vi "Get Command Bits.vi"(8 "error in (no error)":errorcluster, 11 "RFFE RegWrite Command in":refnum<class "RFFE RegWrite Command.lvclass">) -> (0 "error out":errorcluster, 2 "Command Bits":u8[](array[numeric]) format="%02x", 3 "RFFE RegWrite Command out":refnum<class "RFFE RegWrite Command.lvclass">)   [LabVIEW 2018, in "MIPI RFFE API.lvlib" / "RFFE RegWrite Command.lvclass"]
uses:
  RFFE RegWrite Command.lvclass
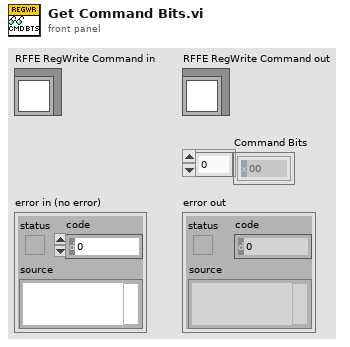
[diagram p1: front panel]
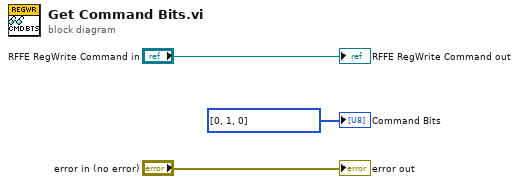
[diagram p0: block diagram]
diagram:
  "error out" <- "error in (no error)"
  "RFFE RegWrite Command out" <- "RFFE RegWrite Command in"
  "Command Bits" <- u8[] [0, 1, 0] ("Command Bits")
